vi "WriteData.vi"(9 "Port Data":u8, 10 "Port name":string, 11 "Reference ID":u64) -> (0 "Error code":i32, 3 "Reference ID out":u64)   [LabVIEW 2023]
doc: "Write channel data to the specified channel"
uses:
  <vilib>/Utility/error.llb/Error Cluster From Error Code.vi
  <vilib>/rvi/errors/niLvFpgaAdjustHostInterfaceError.vi
  <vilib>/rvi/interface/nirviReadWriteControl/nirviReadWriteControl.xnode
  <vilib>/rvi/interface/Simulation/niFpgaSimulationCallBeginRW.vi
  NiFpgaLv.dll
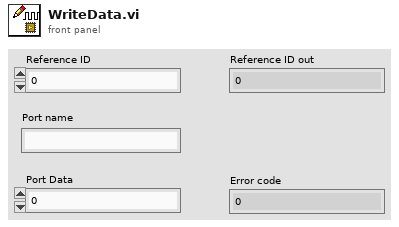
[diagram p1: front panel]
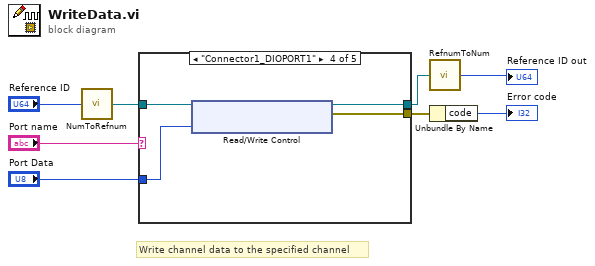
[diagram p0: block diagram]
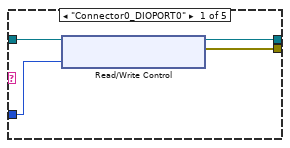
[diagram p2: hidden frame]
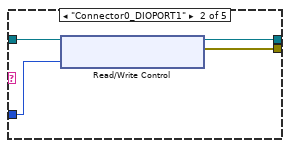
[diagram p3: hidden frame]
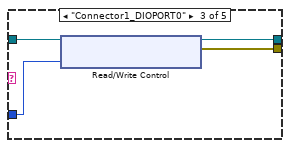
[diagram p4: hidden frame]
diagram:
  # "Write channel data to the specified channel"
  n1 = call "NumToRefnum.vi"("Reference ID"="Reference ID") -> ("Refnum Out"=w8:refnum<k20>)
  n2 = case shown="\"Connector1_DIOPORT1\"" "Port name" {
    tunnel: w8 -> [w12 w16 w20 w24 w25]
    tunnel: [w11 w15 w19 w23 w25] -> w7
    tunnel: [w10 w14 w18 w22 _] -> w6
    tunnel: "Port Data" -> [w9 w13 w17 w21 _]
    frame "Connector0_DIOPORT0" {
      n3 = xnode ("Read/Write Control")("FPGA VI Reference In"=w12, "Connector 0/DIOPORT0"=w9) -> ("FPGA VI Reference Out"=w11:refnum<k20>, "error out"=w10:errorcluster)  [unwired: 1 in]
    }
    frame "Connector0_DIOPORT1" {
      n4 = xnode ("Read/Write Control")("FPGA VI Reference In"=w16, "Connector 0/DIOPORT1"=w13) -> ("FPGA VI Reference Out"=w15:refnum<k20>, "error out"=w14:errorcluster)  [unwired: 1 in]
    }
    frame "Connector1_DIOPORT0" {
      n5 = xnode ("Read/Write Control")("FPGA VI Reference In"=w20, "Connector1/DIOPORT0"=w17) -> ("FPGA VI Reference Out"=w19:refnum<k20>, "error out"=w18:errorcluster)  [unwired: 1 in]
    }
    frame "Connector1_DIOPORT1" {
      n6 = xnode ("Read/Write Control")("FPGA VI Reference In"=w24, "Connector1/DIOPORT1"=w21) -> ("FPGA VI Reference Out"=w23:refnum<k20>, "error out"=w22:errorcluster)  [unwired: 1 in]
    }
    frame Default {
    }
  }
  n7 = call "RefnumToNum.vi"("Refnum in"=w7) -> ("Reference ID"=→"Reference ID out":u64)
  n8 = Unbundle By Name(w6) -> ("code"=→"Error code":i32)
